vi "ConfigureChannelProperties.vi"(8 "error in (no error)":errorcluster, 9 "Sampling Rate":dbl format="%#_13g", 10 "Filtered Channels (in acquisition order)":T5[](array[typedef])) -> (0 "error out":errorcluster, 1 "Tach Config X3":T4[](array[typedef]), 2 "Channel Config X24":T2 {"InputConfig" items=["AC Coupled", "DC Coupled", "IEPE AC Coupled"]}, 3 "Sampling Info":T1={"Number of Channels"=4, "Sampling Rate"=4.0, "Channels"=[], "Units"=[]})   [LabVIEW 2015]
uses:
  <vilib>/addons/InsightCM/MessageBus/Base/controls/Channel.ctl
  <vilib>/addons/InsightCM/MessageBus/Base/controls/KeyValuePair.ctl
  <vilib>/addons/InsightCM/MessageBus/Base/controls/MetricModel.ctl
  <vilib>/addons/InsightCM/Devices/Shared/AcquireBaseLoop/controls/TachometerConfig.ctl
  <vilib>/addons/InsightCM/Devices/Shared/AcquireBaseLoop/controls/FixedSizeArrays.ctl
  <vilib>/LabVIEW Targets/FPGA/cRIO/shared/nicrio_ModuleControls/nicrio_cRIO-9232_ConfigModeRing.ctl
  <vilib>/addons/InsightCM/Devices/Shared/cRIOWfmAcq/subVIs/RIO Wfm Cust Ctrls/rwfm_SamplingInfo.ctl
  <vilib>/addons/InsightCM/Devices/Shared/AcquireBaseLoop/FpgaAcquisition923x.lvlib
  <vilib>/addons/InsightCM/Devices/Shared/cRIOWfmAcq/cRIOWfmLib.lvlib
  <vilib>/addons/InsightCM/Utilities/PropertyHelpers/PropertyHelpers.lvlib
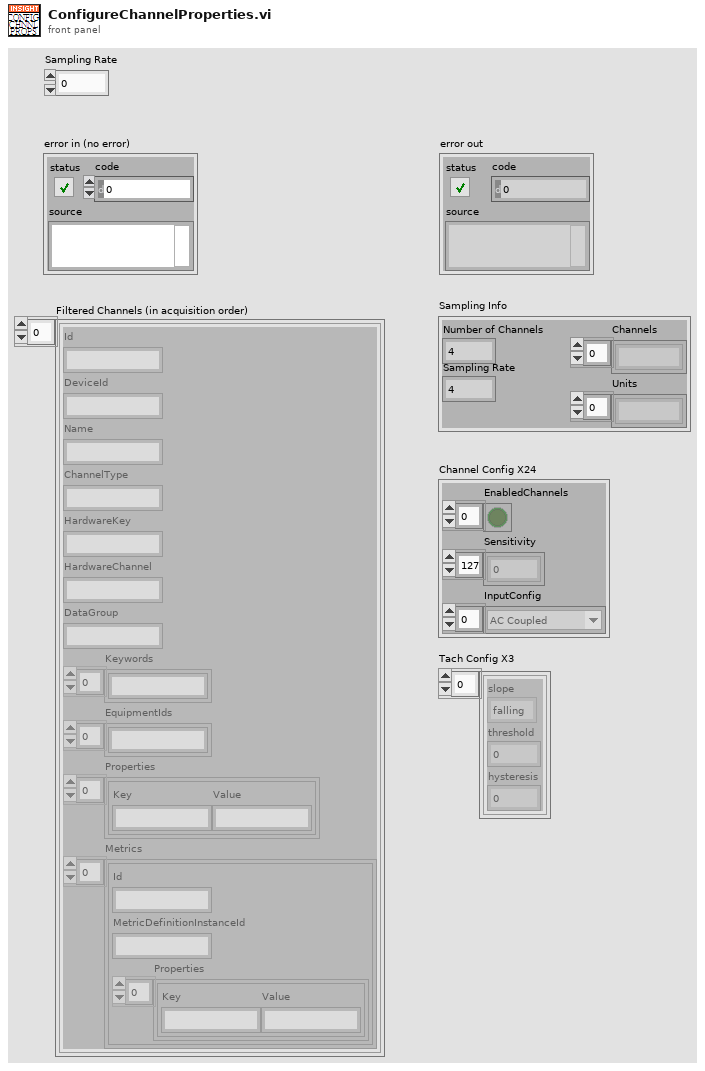
[diagram p1: front panel]
types:
  T1 = typedef "cRIOWfmLib.lvlib/rwfm_SamplingInfo.ctl" = cluster{"Number of Channels":i32, "Sampling Rate":dbl, "Channels":string[], "Units":string[]}
  T2 = typedef "FpgaAcquisition923x.lvlib/FixedSizeArrays.ctl" = cluster{"EnabledChannels":bool[], "Sensitivity":dbl[], "InputConfig":T3[]}
  T3 = typedef "nicrio_cRIO-9232_ConfigModeRing.ctl" = u8
  T4 = typedef "FpgaAcquisition923x.lvlib/TachometerConfig.ctl" = cluster{"slope":enum16{"falling", "rising"}, "threshold":dbl, "hysteresis":dbl}
  T5 = typedef "Channel.ctl" = cluster{"Id":string, "DeviceId":string, "Name":string, "ChannelType":string, "HardwareKey":string, "HardwareChannel":string, "DataGroup":string, "Keywords":string[], "EquipmentIds":string[], "Properties":T6[], "Metrics":T7[]}
  T6 = typedef "KeyValuePair.ctl" = cluster{"Key":string, "Value":string}
  T7 = typedef "MetricModel.ctl" = cluster{"Id":string, "MetricDefinitionInstanceId":string, "Properties":T6[]}
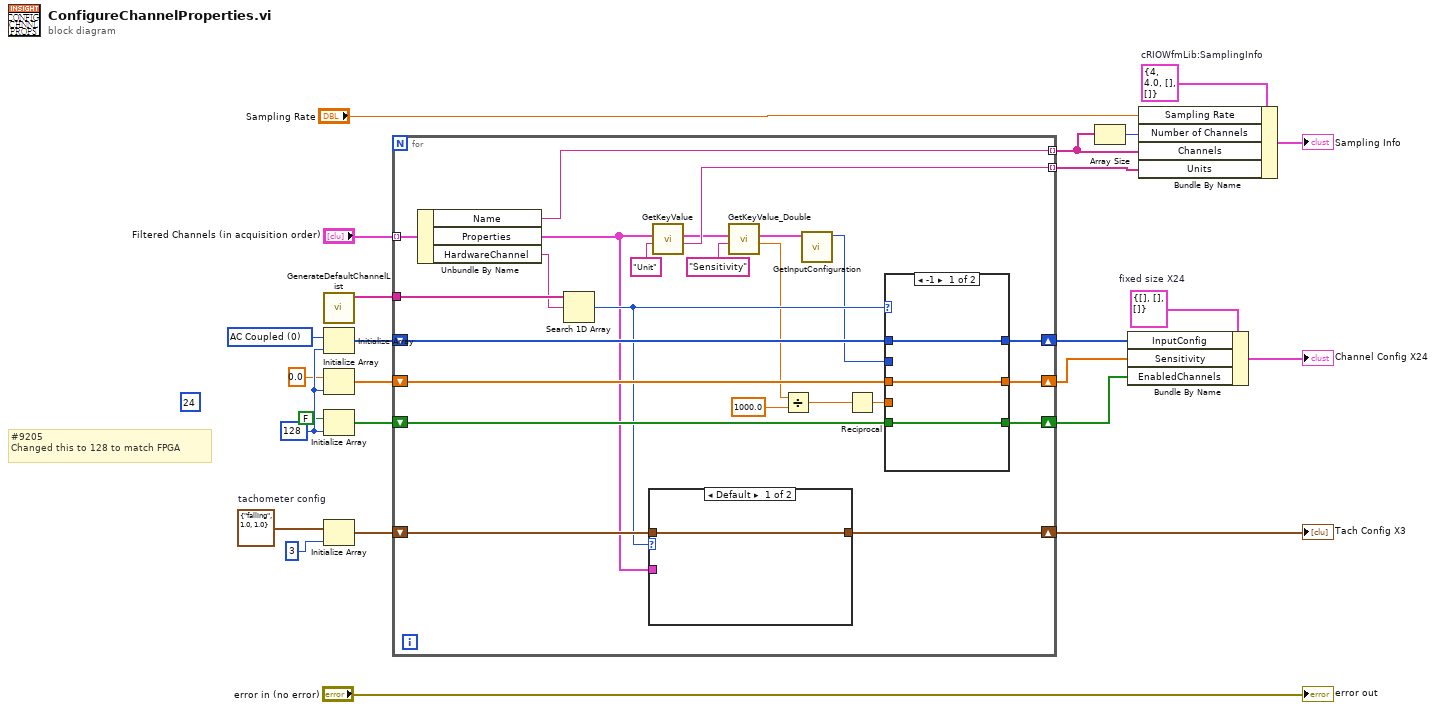
[diagram p0: block diagram]
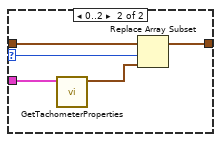
[diagram p2: hidden frame]
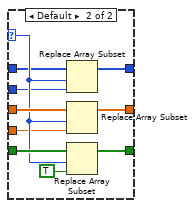
[diagram p3: hidden frame]
diagram:
  (unwired) 24 ("dimension size")
  w7 = T1 {"Number of Channels"=4, "Sampling Rate"=4.0, "Channels"=[], "Units"=[]}  # cRIOWfmLib:SamplingInfo
  w25 = T4 {"slope"=enum."falling", "threshold"=1.0, "hysteresis"=1.0}  # tachometer config
  w18 = T2 {"EnabledChannels"=[], "Sensitivity"=[], "InputConfig"=[]}  # fixed size X24
  w14 = T3 0 items=["AC Coupled", "DC Coupled", "IEPE AC Coupled"] ("Input_Configuration")
  w15 = 128 ("dimension size")
  # "#9205\nChanged this to 128 to match FPGA"
  n1 = call <vilib>:"GenerateDefaultChannelList.vi"() -> ("default channel list"=w8:string[])  [unwired: 11 in]
  n2 = Initialize Array(w14, w15) -> (w17:T3[])
  n3 = Initialize Array(0.0 ("value"), w15) -> (w16:dbl[])
  n4 = Initialize Array(FALSE, w15) -> (w12:bool[])
  n5 = Initialize Array(w25, 3 ("dimension size")) -> (w10:T4[])
  n6 = for {
    tunnel: "Filtered Channels (in acquisition order)" -> [w41] mode=indexing
    shift-right: [w48] -> w21
    shift-left: w12 -> [w49]
    shift-right: [w46] -> w23
    shift-left: w10 -> [w47]
    shift-right: [w44] -> w20
    shift-left: w16 -> [w45]
    shift-right: [w42] -> w19
    shift-left: w17 -> [w43]
    tunnel: w8 -> [w40]
    tunnel: [w38] -> w4 mode=indexing
    tunnel: [w30] -> w6 mode=indexing
    n7 = Unbundle By Name(w41) -> ("Name"=w38:string, "Properties"=w32:T6[], "HardwareChannel"=w39:string)
    n8 = Search 1D Array(1D array=w40, element=w39) -> (index of element=w37:i32)  [unwired: 1 in]
    n9 = case shown="Default" w37 {
      selector: w37 -> [_ w54]
      tunnel: w47 -> [w50 w55]
      tunnel: [w50 w53] -> w46
      tunnel: w32 -> [_ w52]
      frame Default {
      }
      frame 0..2 {
        n10 = call <vilib>:"GetTachometerProperties.vi"("Properties"=w52) -> ("Tachometer Config"=w51:T4)  [unwired: 9 in, 1 out]
        n11 = Replace Array Subset(array=w55, new element=w51, index=w54) -> (w53:T4[])
      }
    }
    n12 = call <vilib>:"GetKeyValue.vi"("key"="Unit" ("name"), "key value pairs"=w32) -> ("value"=w30:string, "key value pairs out"=w29:T6[])  [unwired: 7 in, 1 out]
    n13 = call <vilib>:"GetKeyValue_Double.vi"("key"="Sensitivity" ("name"), "key value pairs"=w29) -> ("value"=w27:dbl, "key value pairs out"=w26:T6[])  [unwired: 7 in, 1 out]
    n14 = Divide(x=w27, y=1000.0) -> (x/y=w34:dbl)
    n15 = call <vilib>:"GetInputConfiguration.vi"("Properties"=w26) -> ("Input Configuration"=w36:T3)  [unwired: 10 in]
    n16 = Reciprocal(x=w34) -> (1/x=w33:dbl)
    n17 = case shown="-1" w37 {
      selector: w37 -> [_ w64]
      tunnel: w49 -> [w58 w68]
      tunnel: [w58 w66] -> w48
      tunnel: w45 -> [w56 w65]
      tunnel: [w56 w63] -> w44
      tunnel: w43 -> [w57 w62]
      tunnel: [w57 w61] -> w42
      tunnel: w36 -> [_ w60]
      tunnel: w33 -> [_ w59]
      frame -1 {
      }
      frame Default {
        n18 = Replace Array Subset(array=w62, new element=w60, index=w64) -> (w61:T3[])
        n19 = Replace Array Subset(array=w65, new element=w59, index=w64) -> (w63:dbl[])
        n20 = Replace Array Subset(array=w68, new element=TRUE, index=w64) -> (w66:bool[])
      }
    }
  }
  "Tach Config X3" <- w23
  n21 = Array Size(array=w4) -> (size(s)=w3:i32)
  n22 = Bundle By Name(cluster=w18, "InputConfig"=w19, "Sensitivity"=w20, "EnabledChannels"=w21) -> (→"Channel Config X24":T2)
  n23 = Bundle By Name(cluster=w7, "Sampling Rate"="Sampling Rate", "Number of Channels"=w3, "Channels"=w4, "Units"=w6) -> (→"Sampling Info":T1)
  "error out" <- "error in (no error)"
